vi "Camera.vi"() -> (0 "Time Out (ms) 2":u8, 1 "Camera 2":bool, 2 "Feature name":string, 3 "Out":bool)   [LabVIEW 2015]
uses:
  Control Button/Exit.ctl
  Feature list/Control PB/Next_.ctl
panel:
  in  "Camera":bool
  in  "Time Out (ms)":u8
  in  "Feature list":string(combo)="Ionizer"
  in  "Next":T1
  in  "Exit":T2
  # "Add Feature List"
  # "CAM1"
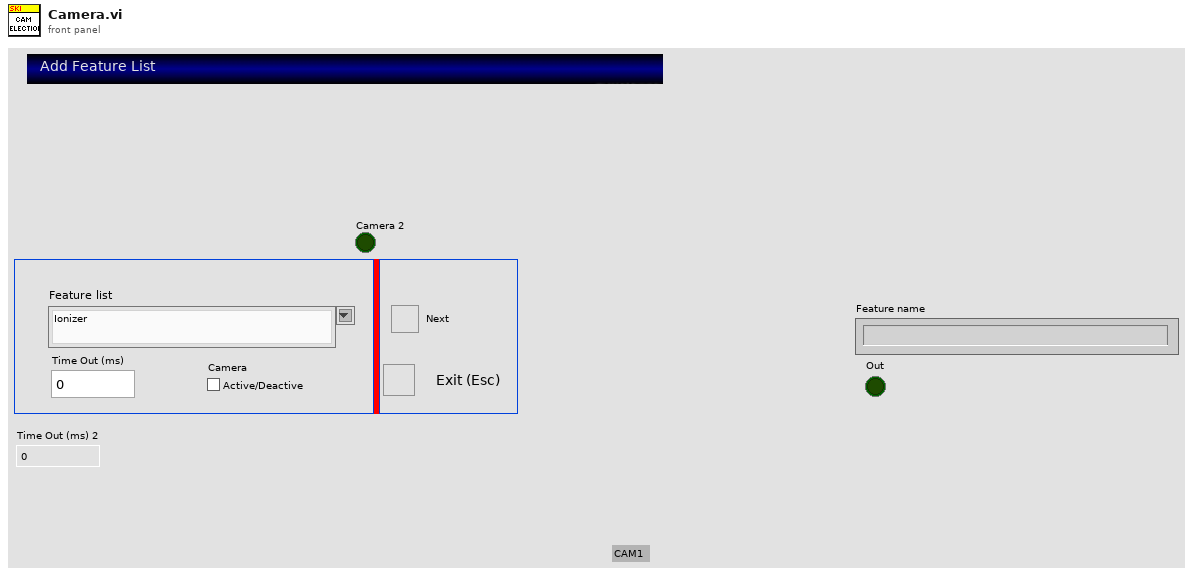
[diagram p1: front panel]
types:
  T1 = typedef "Next_.ctl" = bool
  T2 = typedef "Exit.ctl" = bool
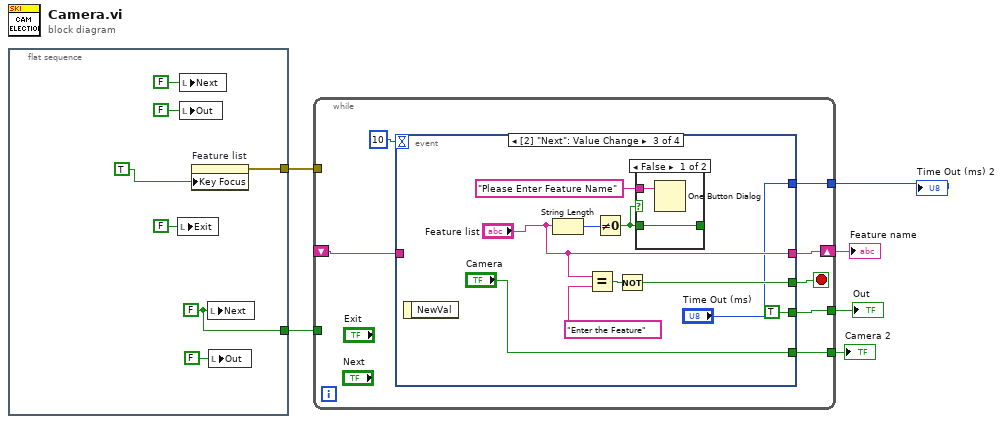
[diagram p0: block diagram]
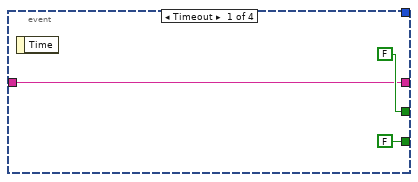
[diagram p2: hidden frame]
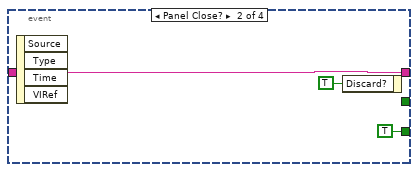
[diagram p3: hidden frame]
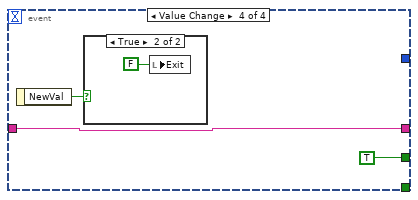
[diagram p5: hidden frame]
diagram:
  n1 = flat-sequence {
    tunnel: [w10] -> w4
    tunnel: [w7] -> w3
    frame #0 {
      w10 = T1 FALSE ("Next")
      n2 = local write "Exit"(FALSE ("Exit")) -> ()
      n3 = local write "Next"(T1 FALSE ("Next")) -> ()
      n4 = local write "Out"(FALSE ("Out")) -> ()
      n5 = property on="Feature list" class="CmbBox"("Key Focus"=TRUE) -> (error out=w7:errorcluster)  [unwired: 2 in, 1 out]
      n6 = local write "Next"(w10) -> ()
      n7 = local write "Out"(FALSE ("Out")) -> ()
    }
  }
  n8 = while {
    tunnel: [w18] -> w5
    tunnel: w4 -> [_]
    shift-right: [w19] -> w6
    shift-left: _ -> [w16]
    tunnel: w3 -> [_]
    tunnel: [w15] -> w2
    tunnel: [w14] -> w1
    stop <- w20 stop-if-true
    n9 = event shown="[2] \"Next\": Value Change" {
      selector: _ -> [_ _ _ _]
      dyn-events: _ -> [_ _ _ _]
      timeout: 10 -> [_ _ _ _]
      tunnel: [FALSE _ w31 TRUE] -> w20
      tunnel: [w21 w24 "Feature list" w40] -> w19
      tunnel: [T1 FALSE ("NewVal") T1 TRUE ("NewVal") T1 TRUE ("NewVal") _] -> w18
      tunnel: w16 -> [w21 w24 _ w40]
      tunnel: [_ _ "Time Out (ms)" _] -> w15
      tunnel: [_ _ "Camera" _] -> w14
      event Timeout {
        n10 = event-data() -> ()  [unwired: 1 in, 1 out]
      }
      event Panel Close? {
        n11 = event-data() -> ()  [unwired: 1 in, 4 out]
        n12 = event-data("Discard?"=TRUE) -> ()  [unwired: 1 in, 1 out]
      }
      event Value Change {
        n13 = event-data() -> ()  [unwired: 1 in, 1 out]
        n14 = String Length(string="Feature list") -> (length=w36:i32)
        n15 = Equal?(x="Feature list", y="Enter the Feature") -> (x = y?=w32:bool)
        n16 = Not Equal To 0?(x=w36) -> (x != 0?=w34:bool)
        n17 = Not(x=w32) -> (.not. x?=w31:bool)
        n18 = case shown="False" w34 {
          tunnel: "Please Enter Feature Name" ("message") -> [w38 _]
          tunnel: [w37 w39] -> _
          tunnel: w34 -> [w37 w39]
          frame False {
            n19 = One Button Dialog(message=w38) -> ()  [unwired: 1 in, 1 out]
          }
          frame True {
          }
        }
      }
      event Value Change {
        n20 = event-data() -> ("NewVal"=w41:T2)  [unwired: 1 in]
        n21 = case shown="True" w41 {
          frame False {
          }
          frame True {
            n22 = local write "Exit"(T1 FALSE ("Next")) -> ()
          }
        }
      }
    }
  }
  "Feature name" <- w6
  "Out" <- w5
  "Time Out (ms) 2" <- w2
  "Camera 2" <- w1
